vi "MAT Read Matrix Header.vi"(7 "offset in (-1: current position)":i64=-1, 8 "Error In":errorcluster, 11 "Ref Num":refnum<file>) -> (0 "error out":errorcluster, 1 "data offset out":i64, 2 "Matrix Name":string, 3 "Dup Ref Num":refnum<file>, 4 "Real/Complex (0 - Real)":u32, 5 "Matrix Size (rows x cols)":i32[](array[numeric]), 6 "Rep. Code":u32, 9 "element byte size":i32, 10 "next variable offset":i64)   [LabVIEW 2013]
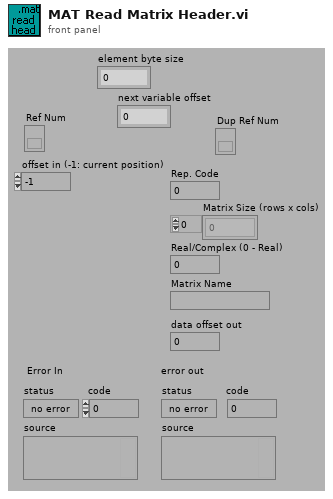
[diagram p1: front panel]
types:
  T1 = enum16{"big-endian, network order", "native, host order", "little-endian"}
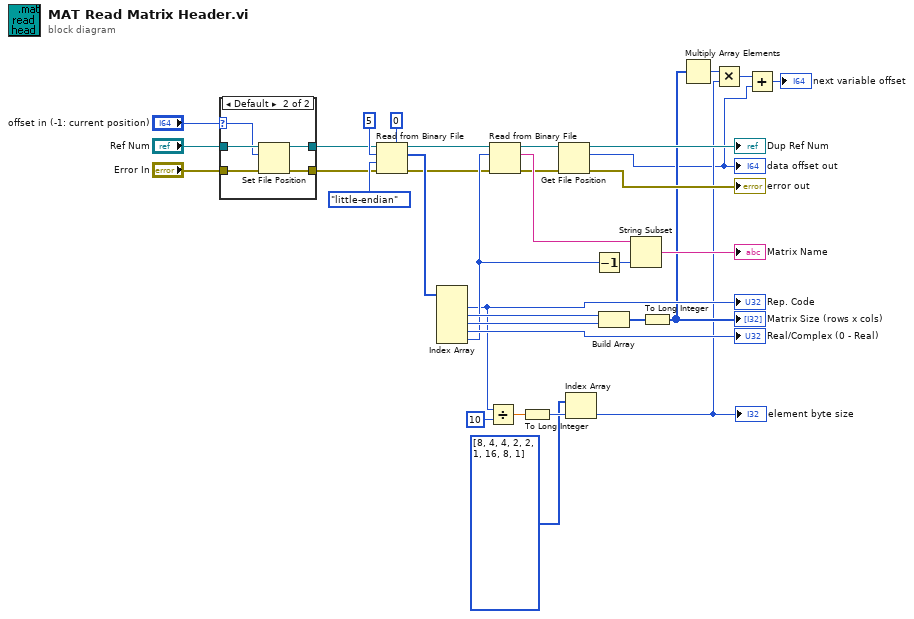
[diagram p0: block diagram]
diagram:
  n1 = case shown="Default" "offset in (-1: current position)" {
    selector: "offset in (-1: current position)" -> [_ w37]
    tunnel: "Error In" -> [w35 w41]
    tunnel: [w35 w40] -> w16
    tunnel: [w36 w39] -> w15
    tunnel: "Ref Num" -> [w36 w38]
    frame -1 {
    }
    frame Default {
      n2 = Set File Position(offset (in bytes) (0)=w37, refnum=w38, error in=w41) -> (refnum out=w39:refnum<file>, error out=w40:errorcluster)  [unwired: 1 in]
    }
  }
  n3 = Read from Binary File(5:u32 0, 8:w16, 9:T1."little-endian" ("byte order (0:big-endian, network order)"), 10:5 ("count"), 11:w15) -> (0:w18:errorcluster, 2:w19:u32[], 3:w17:refnum<file>)  [unwired: 1 in, 1 out]
  n4 = Index Array(array=w19) -> (element #1=w8:u32, element #2=w33:u32, element #3=w32:u32, element #4=→"Real/Complex (0 - Real)":u32, element #5=w29:u32)  [unwired: 5 in]
  "Rep. Code" <- w8
  n5 = Divide(x=w8, y=u32 10) -> (x/y=w10:dbl)
  n6 = Read from Binary File(8:w18, 10:w29, 11:w17) -> (0:w22:errorcluster, 2:w27:string, 3:w23:refnum<file>)  [unwired: 3 in, 1 out]
  n7 = To Long Integer(number=w10) -> (32bit integer=w9:i32)
  n8 = Get File Position(4:w22, 7:w23) -> (0:→"error out":errorcluster, 2:w2:i64, 3:→"Dup Ref Num":refnum<file>)
  "data offset out" <- w2
  n9 = Index Array(array=i32[] [8, 4, 4, 2, 2, 1, 16, 8, 1], index=w9) -> (element=w4:i32)
  "element byte size" <- w4
  n10 = Decrement(x=w29) -> (x-1=w28:u32)
  n11 = Build Array(w33, w32) -> (w31:u32[])
  n12 = String Subset(string=w27, length (rest)=w28) -> (substring=→"Matrix Name":string)  [unwired: 1 in]
  n13 = To Long Integer(number=w31) -> (32bit integer=w6:i32[])
  "Matrix Size (rows x cols)" <- w6
  n14 = Multiply Array Elements(1:w6) -> (0:w5:i32)
  n15 = Multiply(x=w5, y=w4) -> (x*y=w3:i32)
  n16 = Add(x=w3, y=w2) -> (x+y=→"next variable offset":i64)
